vi "Append_Zero_Point_to_End_Array-1.vi"(1 "[IN] Array with \nDisplacements":dbl[](array[numeric])) -> (0 "[OUT] Array with \nAppended Point":dbl[](array[numeric]))   [LabVIEW 2017]
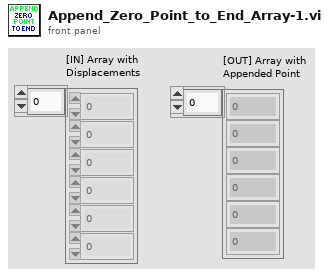
[diagram p1: front panel]
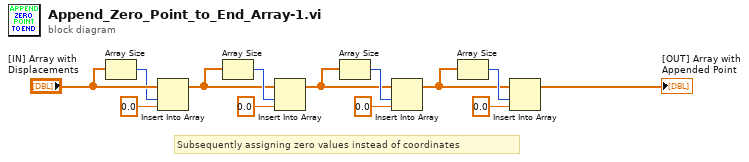
[diagram p0: block diagram]
diagram:
  # "Subsequently assigning zero values instead of coordinates"
  n1 = Array Size(array="[IN] Array with \nDisplacements") -> (size(s)=w11:i32)
  n2 = Insert Into Array(array="[IN] Array with \nDisplacements", index=w11, new element=0.0 ("new element/subarray")) -> (w8:dbl[])
  n3 = Array Size(array=w8) -> (size(s)=w9:i32)
  n4 = Insert Into Array(array=w8, index=w9, new element=0.0 ("new element/subarray")) -> (w5:dbl[])
  n5 = Array Size(array=w5) -> (size(s)=w6:i32)
  n6 = Insert Into Array(array=w5, index=w6, new element=0.0 ("new element/subarray")) -> (w2:dbl[])
  n7 = Array Size(array=w2) -> (size(s)=w3:i32)
  n8 = Insert Into Array(array=w2, index=w3, new element=0.0 ("new element/subarray")) -> (→"[OUT] Array with \nAppended Point":dbl[])
